vi "AWG offset.vi"() -> ()   [LabVIEW 2018]
uses:
  <instrlib>/Tektronix AWG 5000 7000 Series/Tektronix AWG 5000 7000 Series.lvlib
panel:
  in  "error in (no error)":errorcluster
  in  "VISA resource name":refnum<visa-resource-name>="GPIB0::1::INSTR"
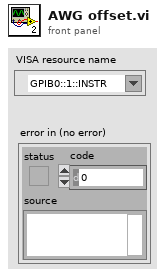
[diagram p1: front panel]
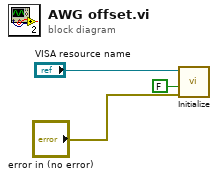
[diagram p0: block diagram]
diagram:
  n1 = call <instrlib>:"Initialize.vi"("error in (no error)"="error in (no error)", "Reset (False)"=FALSE ("Reset? (F: No)"), "VISA resource name"="VISA resource name") -> ()  [unwired: 7 in, 2 out]
